vi "PathPlanner_Path_BezierToWaypoints.vi"(11 "BezierPoints":T1[](array[typedef]) {"Y" format="%14.3f"; "X" format="%14.3f"}) -> (3 "waypoints":T2(array[cluster]))   [LabVIEW 2019, in "PathPlanner24.lvlib"]
doc: "Convert bezier points to waypoints allowing them to be written to a JSON string.\n\nInputs: \n - Bezier - array of translation2s - List of bezier points\n\nOutputs:\n - waypoints - array of cluster - waypoints compatible with pathplanner path JSON strings."
uses:
  PathPlanner24.lvlib
  <vilib>/Rock Robotics/WPI/ThirdParty/JAS_Junk/TrajLib/TypeDef/TRANSLATION2D.ctl
  <vilib>/Rock Robotics/WPI/ThirdParty/JAS_Junk/TrajLib/Trajectory_Library.lvlib
panel:
  in  "waypoints":T3={"anchor"={"x"=1e+30, "y"=1e+31}, "prevControl"={"x"=1e+30, "y"=1e+31}, "nextControl"={"x"=1e+30, "y"=1e+31}, "isLocked"=FALSE}
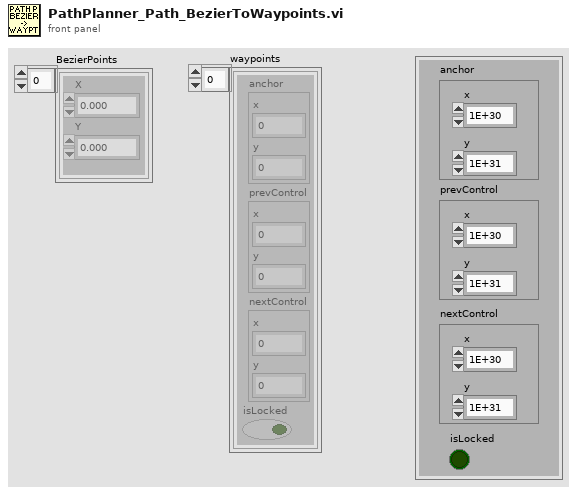
[diagram p1: front panel]
types:
  T1 = typedef "Trajectory_Library.lvlib/TRANSLATION2D.ctl" = cluster{"X":dbl, "Y":dbl}
  T2 = cluster{"anchor":cluster{"x":dbl, "y":dbl}, "prevControl":cluster{"x":dbl, "y":dbl}, "nextControl":cluster{"x":dbl, "y":dbl}, "isLocked":bool}[]
  T3 = cluster{"anchor":cluster{"x":dbl, "y":dbl}, "prevControl":cluster{"x":dbl, "y":dbl}, "nextControl":cluster{"x":dbl, "y":dbl}, "isLocked":bool}
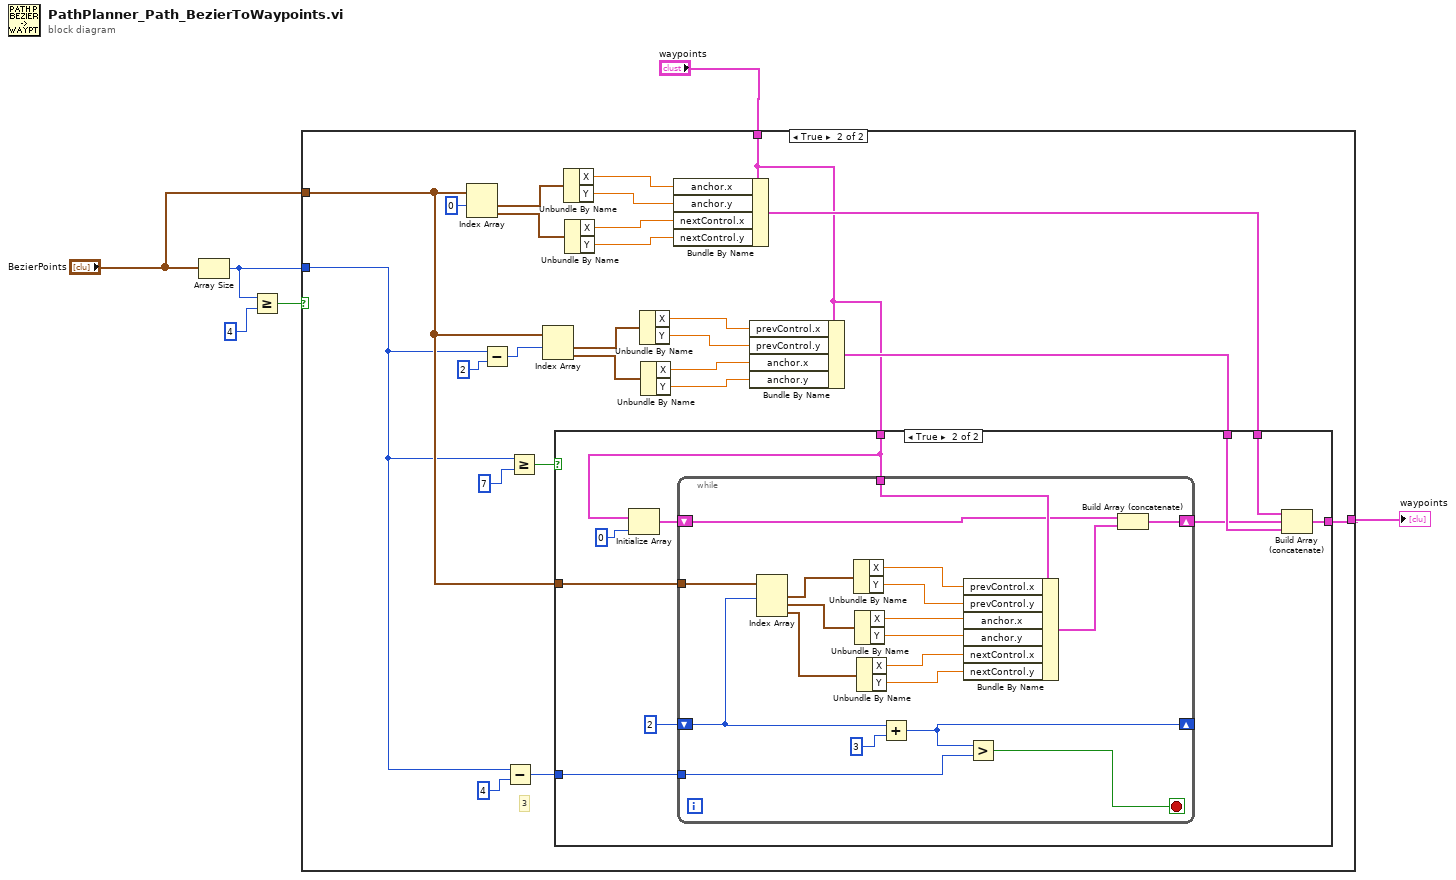
[diagram p0: block diagram]
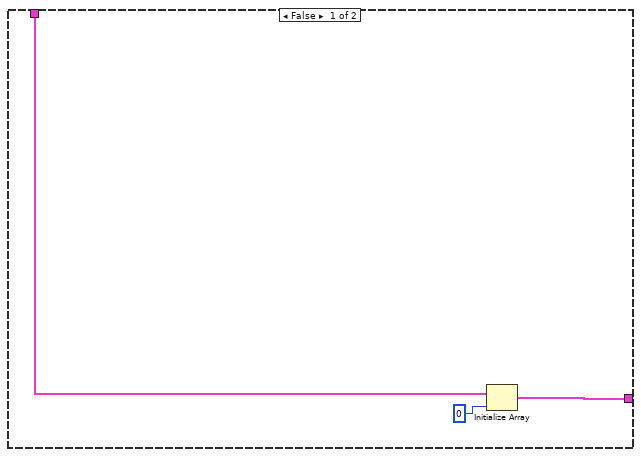
[diagram p2: hidden frame]
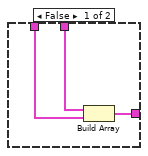
[diagram p3: hidden frame]
diagram:
  n1 = Array Size(array="BezierPoints") -> (size(s)=w2:i32)
  n2 = Greater Or Equal?(x=w2, y=4) -> (x >= y?=w3:bool)
  n3 = case shown="True" w3 {
    tunnel: "waypoints" -> [w8 w14]
    tunnel: "BezierPoints" -> [_ w13]
    tunnel: w2 -> [_ w12]
    tunnel: [w7 w15] -> w1
    frame False {
      n4 = Initialize Array(w8, 0 ("dimension size")) -> (w7:T2)
    }
    frame True {
      # "3"
      n5 = Index Array(array=w13, index #1=0 ("index")) -> (element #1=w33:T1, element #2=w32:T1)  [unwired: 1 in]
      n6 = Subtract(x=w12, y=2) -> (x-y=w20:i32)
      n7 = Subtract(x=w12, y=4) -> (x-y=w10:i32)
      n8 = Greater Or Equal?(x=w12, y=7) -> (x >= y?=w18:bool)
      n9 = Index Array(array=w13, index #1=w20) -> (element #1=w27:T1, element #2=w26:T1)  [unwired: 1 in]
      n10 = Unbundle By Name(w33) -> ("X"=w31:dbl, "Y"=w30:dbl)
      n11 = Unbundle By Name(w32) -> ("X"=w29:dbl, "Y"=w28:dbl)
      n12 = Unbundle By Name(w27) -> ("X"=w25:dbl, "Y"=w24:dbl)
      n13 = Unbundle By Name(w26) -> ("X"=w23:dbl, "Y"=w22:dbl)
      n14 = Bundle By Name(cluster=w14, "anchor.x"=w31, "anchor.y"=w30, "nextControl.x"=w29, "nextControl.y"=w28) -> (w17:T3)
      n15 = Bundle By Name(cluster=w14, "prevControl.x"=w25, "prevControl.y"=w24, "anchor.x"=w23, "anchor.y"=w22) -> (w16:T3)
      n16 = case shown="True" w18 {
        tunnel: w17 -> [w37 w40]
        tunnel: w16 -> [w36 w39]
        tunnel: [w35 w41] -> w15
        tunnel: w14 -> [_ w44]
        tunnel: w13 -> [_ w43]
        tunnel: w10 -> [_ w42]
        frame False {
          n17 = Build Array(w37, w36) -> (w35:T2)
        }
        frame True {
          n18 = Initialize Array(w44, 0 ("dimension size")) -> (w45:T2)
          n19 = while {
            shift-right: [w51] -> _
            shift-left: 2 ("y") -> [w53]
            shift-right: [w48] -> w38
            shift-left: w45 -> [w55]
            tunnel: w44 -> [w66]
            tunnel: w43 -> [w65]
            tunnel: w42 -> [w50]
            stop <- w49 stop-if-true
            n20 = Index Array(array=w65, index #1=w53) -> (element #1=w64:T1, element #2=w63:T1, element #3=w62:T1)  [unwired: 2 in]
            n21 = Unbundle By Name(w64) -> ("X"=w61:dbl, "Y"=w60:dbl)
            n22 = Unbundle By Name(w63) -> ("X"=w59:dbl, "Y"=w58:dbl)
            n23 = Unbundle By Name(w62) -> ("X"=w57:dbl, "Y"=w56:dbl)
            n24 = Add(x=w53, y=3) -> (x+y=w51:i32)
            n25 = Bundle By Name(cluster=w66, "prevControl.x"=w61, "prevControl.y"=w60, "anchor.x"=w59, "anchor.y"=w58, "nextControl.x"=w57, "nextControl.y"=w56) -> (w54:T3)
            n26 = Greater?(x=w51, y=w50) -> (0:w49:bool)
            n27 = Build Array (concatenate)(w55, w54) -> (w48:T2)
          }
          n28 = Build Array (concatenate)(w40, w38, w39) -> (w41:T2)
        }
      }
    }
  }
  "waypoints" <- w1
